vi "Destroy.vi"(8 "error in (no error)":errorcluster, 11 "publisher":refnum<class "IcmMessagePublisher.lvclass">) -> (0 "error out":errorcluster)   [LabVIEW 2017, in "IcmMessagePublisher.lvclass"]
doc: "Ends the message-bus session for a particular service."
uses:
  <vilib>/addons/InsightCM/MessageBus/MessagePublisher/IcmMessagePublisher.lvclass
  <vilib>/addons/InsightCM/MessageBus/MessagePublisher/IcmMessagePublisher.lvclass/IcmMessagePublisher.ctl
  C:/Program Files (x86)/National Instruments/LabVIEW 2017/vi.lib/addons/InsightCM/Binaries/LabviewMessageAdapter.dll
  Binaries/LabviewMessageAdapter.dll
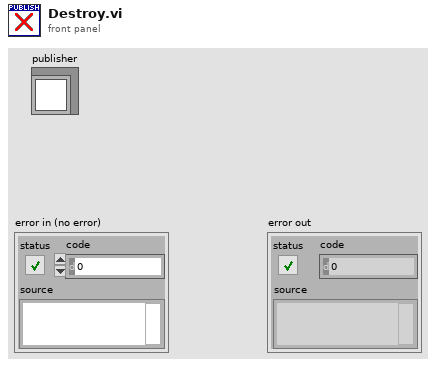
[diagram p1: front panel]
types:
  T1 = typedef "MessagePublisherDvr.ctl" = refnum<data-value>
  T2 = typedef "MessagePublisherData.ctl" = cluster{"Publisher":refnum<k24>}
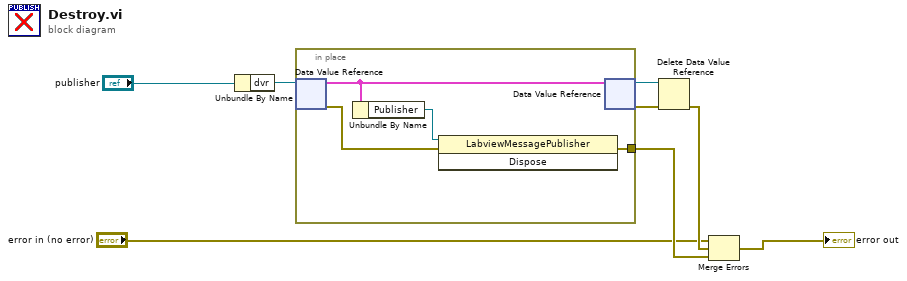
[diagram p0: block diagram]
diagram:
  n1 = Unbundle By Name("publisher") -> ("dvr"=w6:T1)
  n2 = in-place {
    in-place-border: [w9] -> w5
    n3 = in-place-dvr #1(w6) -> (w12:T2, w10:errorcluster)
    n4 = Unbundle By Name(w12) -> ("Publisher"=w11:refnum<k24>)
    n5 = invoke class="LabviewMessagePublisher" method="Dispose"(reference=w11, error in=w10) -> (error out=w9:errorcluster)  [unwired: 1 in, 2 out]
    n6 = in-place-dvr #1(w12) -> (w2:T1, w4:errorcluster)
  }
  n7 = Delete Data Value Reference(data value reference=w2, error in=w4) -> (error out=w3:errorcluster)  [unwired: 1 out]
  n8 = Merge Errors("error in (no error)", w3, w5) -> (→"error out":errorcluster)
